vi "FTW-SQLite-CloseConnection.vi"(0 "SQLite Connector":refnum<class "FTW-SQLite-Connector.lvclass">, 11 "error in":errorcluster) -> (15 "error out":errorcluster)   [LabVIEW 2013, in "FTW-SQLite-Connector.lvclass"]
uses:
  FTW-SQLite-Connector.lvclass
  FTW-SQLite-Connector.lvclass/FTW-SQLite-Connector.ctl
panel:
  # "Inputs"
  # "Outputs"
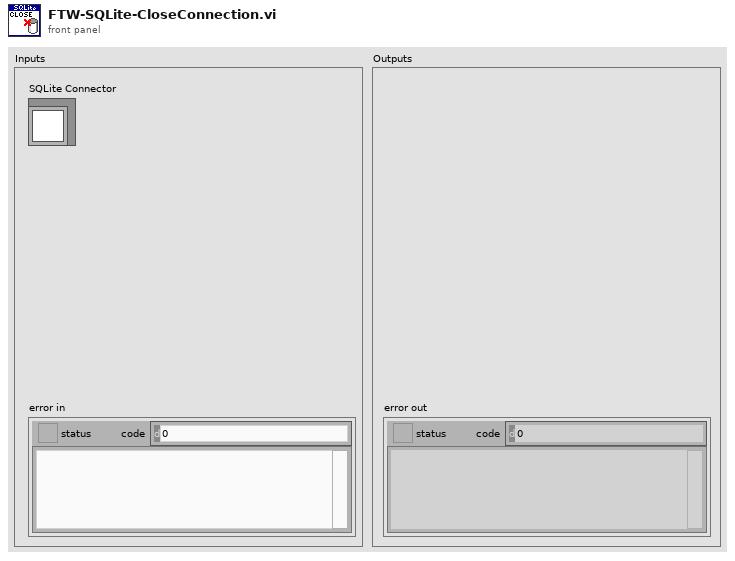
[diagram p1: front panel]
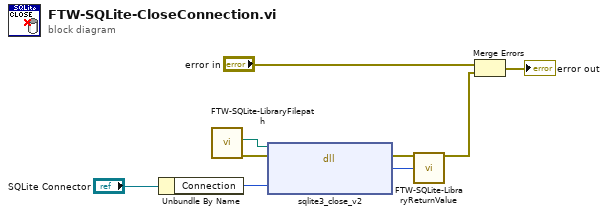
[diagram p0: block diagram]
diagram:
  n1 = Unbundle By Name("SQLite Connector") -> ("Connection"=w4:u64)
  n2 = call "FTW-SQLite-LibraryFilepath.vi"() -> ("error out"=w7:errorcluster, "SQLite Library Filepath"=w6:path)  [unwired: 9 in, 1 out]
  n3 = dll-call lib="?" fn="sqlite3_close_v2"(path in=w6, error in=w7, "Connection Handle"=w4) -> (error out=w9:errorcluster, "Return Value"=w8:i32)  [unwired: 2 in, 1 out]
  n4 = call "FTW-SQLite-LibraryReturnValue.vi"("error in"=w9, "Return Value"=w8) -> ("error out"=w2:errorcluster)  [unwired: 13 in]
  n5 = Merge Errors("error in", w2) -> (→"error out":errorcluster)
